vi "VISA IDN M81 Fix.vi"(6 "Manufacturer in":string="Lake Shore", 7 "Revision in":string="ver3.6", 8 "error in (no error)":errorcluster {"code" format="%.0x"}, 9 "Info in":string="s/n130040", 10 "Model in":string="M81-6", 11 "VISA Resource Name":refnum<visa-resource-name>="GPIB0::12::INSTR") -> (0 "error out":errorcluster {"code" format="%.0x"}, 2 "Devices":T1[](array[typedef]) {"Status" format="%.0x"}, 3 "dup VISA Session":refnum<visa-resource-name>)   [LabVIEW 2025]
doc: "Author: Scott Hannahs <sth@magnet.fsu.edu>\n\nThis software is licensed for use under the “MIT License\"\nCopyright (c) 2025 Scott Hannahs, sth@sth@magnet.sthnet.net\n\nPermission is hereby granted, free of charge, to any person obtaining a copy of this software and associated documentation files (the \"Software\"), to deal in the Software without restriction, including without limitation the rights to use, copy, modify, merge, publish, distribute, sublicense, and/or sell copies of the Software, and to permit persons to whom the Software is furnished to do so, subject to the following conditions: The above copyright notice and this permission notice shall be included in all copies or substantial portions of the Software.\n\nTHE SOFTWARE IS PROVIDED \"AS IS\", WITHOUT WARRANTY OF ANY KIND, EXPRESS OR IMPLIED, INCLUDING BUT NOT LIMITED TO THE WARRANTIES OF MERCHANTABILITY, FITNESS FOR A PARTICULAR PURPOSE AND NONINFRINGEMENT. IN NO EVENT SHALL THE AUTHORS OR COPYRIGHT HOLDERS BE LIABLE FOR ANY CLAIM, DAMAGES OR OTHER LIABILITY, WHETHER IN AN ACTION OF CONTRACT, TORT OR OTHERWISE, ARISING FROM, OUT OF OR IN CONNECTION WITH THE SOFTWARE OR THE USE OR OTHER DEALINGS IN THE SOFTWARE."
uses:
  New NML Data Acq/Sub Controls/Instrument IDN.ctl
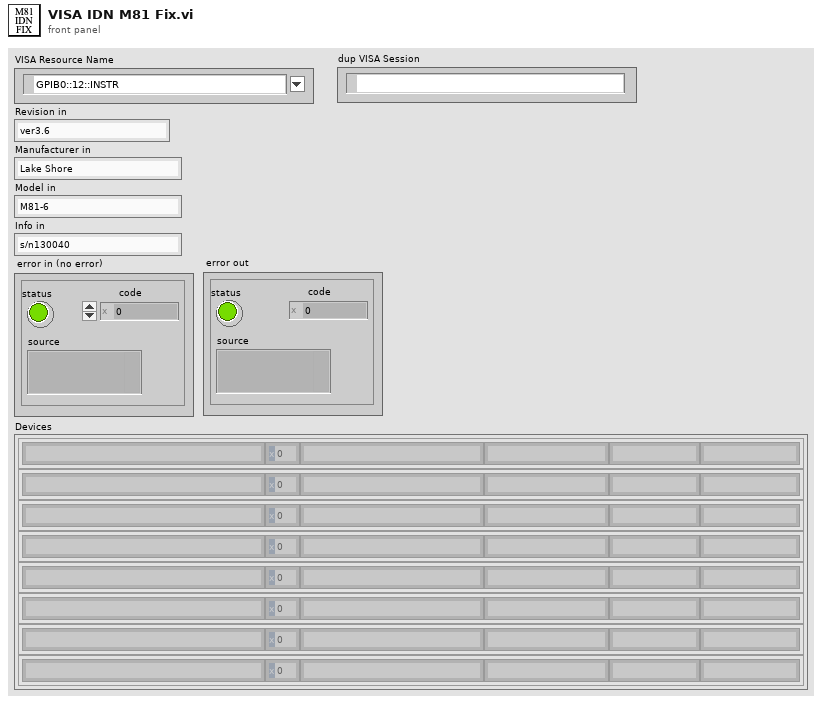
[diagram p1: front panel]
types:
  T1 = typedef "Instrument IDN.ctl" = cluster{"VISA Address":string, "Status":u16, "Manufacturer":string, "Model":string, "Info":string, "Info 2":string, "Misc Data":variant}
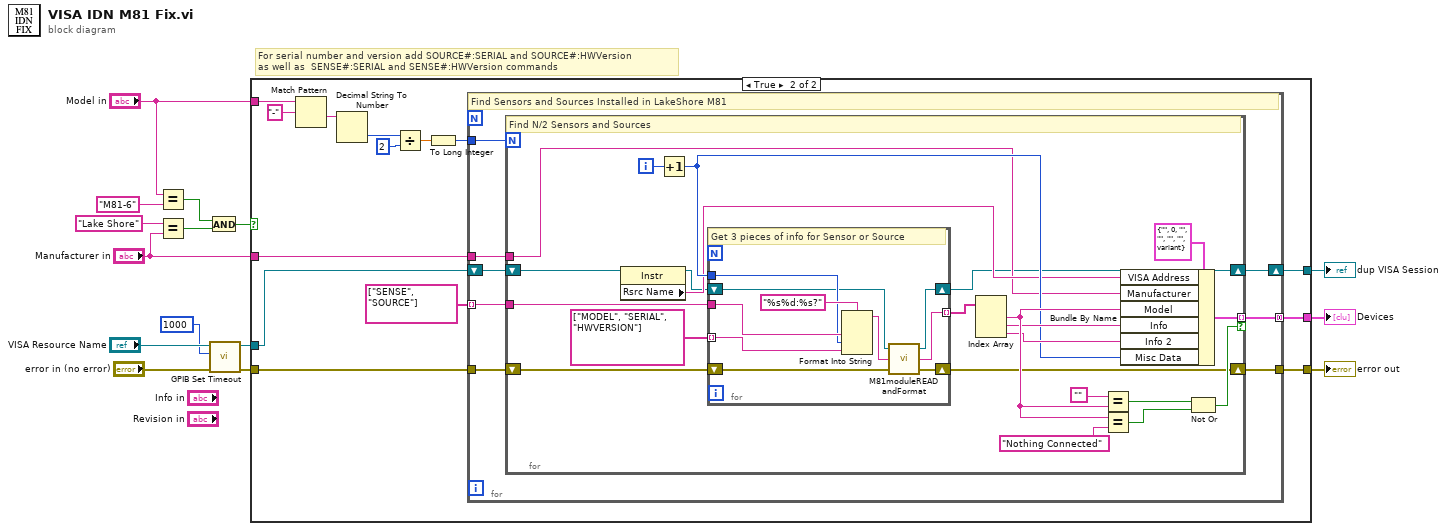
[diagram p0: block diagram]
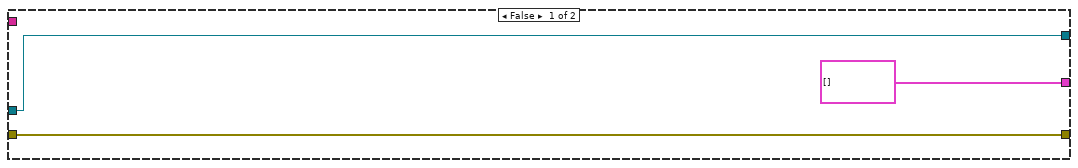
[diagram p2: hidden frame]
diagram:
  # "For serial number and version add SOURCE#:SERIAL and SOURCE#:HWVersion \nas well as  SENSE#:SERIAL and SENSE#:HWVersion commands"
  n1 = Equal?(x="Model in", y="M81-6") -> (x = y?=w9:bool)
  n2 = Equal?(x="Lake Shore" ("y"), y="Manufacturer in") -> (x = y?=w13:bool)
  n3 = And(x=w9, y=w13) -> (x .and. y?=w15:bool)
  n4 = call "GPIB Set Timeout.vi"("Error In"="error in (no error)", "Timeout"=u32 1000, "VISA resource name"="VISA Resource Name") -> ("Error Out"=w2:errorcluster, "dup VISA resource name"=w5:refnum<visa-resource-name>)  [unwired: 2 in, 1 out]
  n5 = case shown="True" w15 {
    tunnel: "Model in" -> [_ w27]
    tunnel: w2 -> [w16 w19]
    tunnel: [T1[] [] w22] -> w4
    tunnel: w5 -> [w17 w23]
    tunnel: [w17 w20] -> w11
    tunnel: "Manufacturer in" -> [_ w24]
    tunnel: [w16 w21] -> w1
    frame False {
    }
    frame True {
      n6 = Match Pattern(string=w27, regular expression="-") -> (after substring=w31:string)  [unwired: 1 in, 3 out]
      n7 = Decimal String To Number(string=w31) -> (number=w29:i32)  [unwired: 2 in, 1 out]
      n8 = Divide(x=w29, y=i8 2) -> (x/y=w28:dbl)
      n9 = To Long Integer(number=w28) -> (32bit integer=w25:i32)
      n10 = for {
        tunnel: string[] ["SENSE", "SOURCE"] -> [w39] mode=indexing
        tunnel: w25 -> [w40]
        tunnel: w24 -> [w38]
        tunnel: [w36] -> w22 mode=concatenating
        tunnel: [w35] -> w21
        shift-right: [w34] -> w20
        shift-left: w23 -> [w37]
        tunnel: w19 -> [w33]
        # "Find Sensors and Sources Installed in LakeShore M81"
        n11 = for {
          N: w40 -> [_]
          tunnel: w38 -> [w46]
          tunnel: w39 -> [w60]
          tunnel: [w54] -> w36 mode=indexing if=w52
          shift-right: [w45] -> w35
          shift-left: w33 -> [w44]
          shift-right: [w42] -> w34
          shift-left: w37 -> [w43]
          i -> [w62]
          # "Find N/2 Sensors and Sources"
          n12 = property class="Instr"(reference=w43) -> (reference out=w41:refnum<visa-resource-name>, "Rsrc Name"=w47:string)  [unwired: 1 in, 1 out]
          n13 = Increment(x=w62) -> (x+1=w48:i32)
          n14 = for {
            tunnel: string[] ["MODEL", "SERIAL", "HWVERSION"] -> [w70] mode=indexing
            tunnel: w60 -> [w69]
            tunnel: w48 -> [w68]
            shift-right: [w67] -> w42
            shift-left: w41 -> [w66]
            shift-right: [w64] -> w45
            shift-left: w44 -> [w65]
            tunnel: [w63] -> w59 mode=indexing
            # "Get 3 pieces of info for Sensor or Source"
            n15 = Format Into String(format string="%s%d:%s?" ("write buffer (\"\")"), w69, w68, w70) -> (resulting string=w71:string)  [unwired: 2 in, 1 out]
            n16 = call "M81moduleREADandFormat.vi"("error in (no error)"=w65, "Command"=w71, "VISA resource name"=w66) -> ("error out"=w64:errorcluster, "result string"=w63:string, "dup VISA Session"=w67:refnum<visa-resource-name>)
          }
          n17 = Index Array(array=w59) -> (element #1=w51:string, element #2=w50:string, element #3=w49:string)  [unwired: 3 in]
          n18 = Equal?(x="", y=w51) -> (x = y?=w55:bool)
          n19 = Equal?(x=w51, y="Nothing Connected") -> (x = y?=w56:bool)
          n20 = Bundle By Name(cluster=T1 {"VISA Address"="", "Status"=0, "Manufacturer"="", "Model"="", "Info"="", "Info 2"="", "Misc Data"=variant} ("Instrument List"), "VISA Address"=w47, "Manufacturer"=w46, "Model"=w51, "Info"=w50, "Info 2"=w49, "Misc Data"=w48) -> (w54:T1)
          n21 = Not Or(1:w56, 2:w55) -> (0:w52:bool)
        }
      }
    }
  }
  "error out" <- w1
  "Devices" <- w4
  "dup VISA Session" <- w11
